vi "get_objects.vi"(0 "HGF_FGV_Clear":refnum<class "HGF_FGV_Clear.lvclass">, 5 "error in (no error)":errorcluster) -> (14 "dup HGF_FGV_Clear":refnum<class "HGF_FGV_Clear.lvclass">, 16 "objects":refnum<class>[](array[class]), 19 "error out":errorcluster)   [LabVIEW 2012, in "HGF_FGV.lvlib" / "HGF_FGV_Clear.lvclass"]
doc: "Returns the objects of FGV DB instance."
uses:
  HGF_FGV_Clear.lvclass
  HGF_FGV_Clear.lvclass/HGF_FGV_Clear.ctl
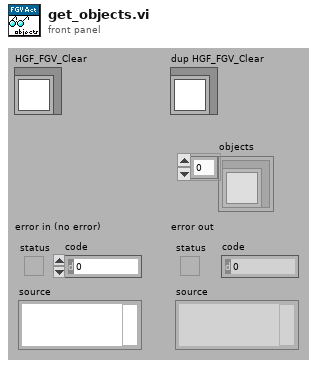
[diagram p1: front panel]
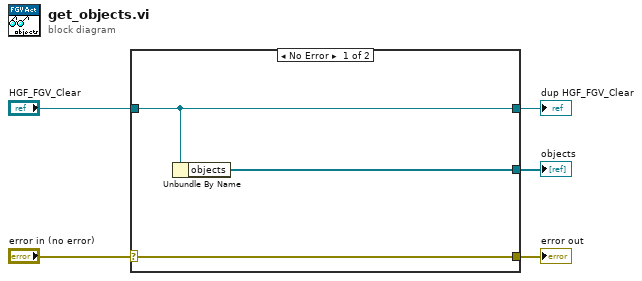
[diagram p0: block diagram]
diagram:
  n1 = case shown="No Error" "error in (no error)" {
    selector: "error in (no error)" -> [w8 w9]
    tunnel: [w8 w9] -> w4
    tunnel: [w7 w10] -> w2
    tunnel: "HGF_FGV_Clear" -> [w7 w10]
    tunnel: [w6 _] -> w1
    frame No Error {
      n2 = Unbundle By Name(w7) -> ("objects"=w6:refnum<class>[])
    }
    frame Error {
    }
  }
  "error out" <- w4
  "dup HGF_FGV_Clear" <- w2
  "objects" <- w1
